vi "configmgr-encoding-test.vi"(8 "error in (no error)":errorcluster) -> (0 "error out":errorcluster)   [LabVIEW 2013]
uses:
  <vilib>/LabVIEW Open Source/Configuration Manager/Encoding/Encoding.lvclass
  <vilib>/LabVIEW Open Source/Configuration Manager/Encoding.Base64/Encoding.Base64.lvclass
  <vilib>/addons/_JKI Toolkits/Caraya/classes/Test/Test.lvclass
  <vilib>/addons/_JKI Toolkits/Caraya/classes/Assert/Assert.lvclass
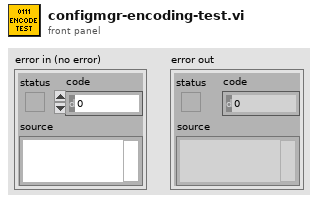
[diagram p1: front panel]
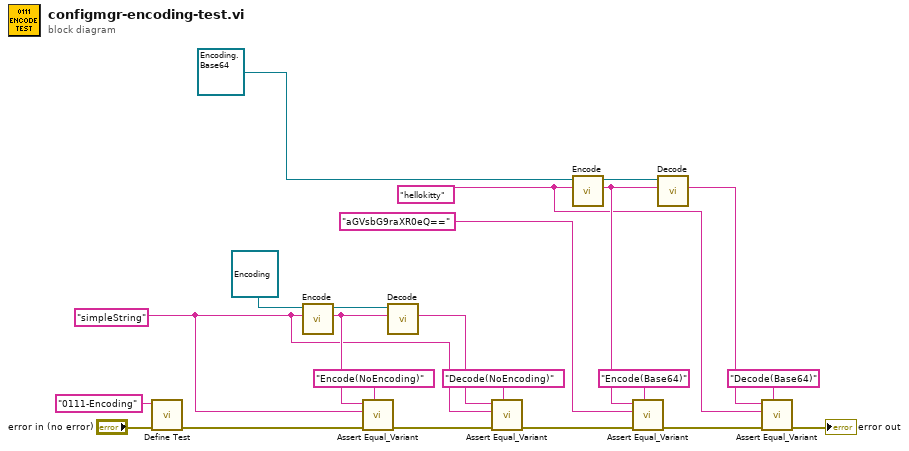
[diagram p0: block diagram]
diagram:
  w6 = "hellokitty" ("Name")
  w3 = "simpleString" ("Name")
  n1 = call <vilib>:"Define Test.vi"("error in (no error)"="error in (no error)", "Label (VI Title)"="0111-Encoding") -> ("error out"=w21:errorcluster)  [unwired: 9 in]
  n2 = call-dynamic "Encode.vi"("String"=w3, "CfgEncoding in"=refnum<class "Encoding.lvclass"> refnum) -> ("Encoded String"=w4:string, "CfgEncoding out"=w18:refnum<class "Encoding.lvclass">)  [unwired: 8 in]
  n3 = call <vilib>:"Assert Equal_Variant.vi"("Label"="Encode(NoEncoding)" ("Label (VI Title)"), "error in (no error)"=w21, "Y"=w3, "X"=w4) -> ("error out"=w16:errorcluster)  [unwired: 7 in]
  n4 = call-dynamic "Decode.vi"("Encoded String"=w4, "CfgEncoding in"=w18) -> ("String"=w15:string)  [unwired: 8 in, 1 out]
  n5 = call <vilib>:"Assert Equal_Variant.vi"("Label"="Decode(NoEncoding)" ("Label (VI Title)"), "error in (no error)"=w16, "Y"=w3, "X"=w15) -> ("error out"=w8:errorcluster)  [unwired: 7 in]
  n6 = call-dynamic "Encode.vi"("String"=w6, "Encoding in"=refnum<class "Encoding.Base64.lvclass"> refnum ("CfgEncoding in")) -> ("Encoded String"=w14:string, "Encoding out"=w10:refnum<class "Encoding.Base64.lvclass">)  [unwired: 8 in]
  n7 = call <vilib>:"Assert Equal_Variant.vi"("Label"="Encode(Base64)" ("Label (VI Title)"), "error in (no error)"=w8, "Y"="aGVsbG9raXR0eQ==" ("Name"), "X"=w14) -> ("error out"=w12:errorcluster)  [unwired: 7 in]
  n8 = call-dynamic "Decode.vi"("Encoded String"=w14, "CfgEncoding in"=w10) -> ("String"=w13:string)  [unwired: 8 in, 1 out]
  n9 = call <vilib>:"Assert Equal_Variant.vi"("Label"="Decode(Base64)" ("Label (VI Title)"), "error in (no error)"=w12, "Y"=w6, "X"=w13) -> ("error out"=→"error out":errorcluster)  [unwired: 7 in]
